vi "Test Copy Array To Image Pixel.vi"(8 "error in (no error)":errorcluster, 11 "Test Case In":refnum<class "Image.lvclass">) -> (0 "error out":errorcluster, 3 "Test Case Out":refnum<class "Image.lvclass">)   [LabVIEW 2020, in "g_ar_toolkit.test.lvlib" / "Image.lvclass"]
uses:
  Image.lvclass
  C:/Program Files (x86)/National Instruments/LabVIEW 2020/vi.lib/Astemes/LUnit/Test Case.lvclass
  g_ar_toolkit.common/Image Size (Integer).ctl
  <vilib>/Astemes/LUnit/Test Case.lvclass/Test Case.ctl
  g_ar_toolkit.image/New Image (ARGB).vi
  4993e8ee-a06a-463a-9684-69129f64d5ce.vi
  b5d9ff70-754c-4220-963e-cc8b9679940b.vi
  g_ar_toolkit.image/Copy Array to Image.vi
  g_ar_toolkit.image/Copy Array to Image (ARGB).vi
  g_ar_toolkit.image/New Image (ARGB).vi/3321fa97-f432-4e1e-8db9-a0df79aed21b.vi
  g_ar_toolkit.image/ARGB Colour to U32 Pixel Value.vi
  <vilib>/Astemes/LUnit/Append Pass Result.vi
  <vilib>/Astemes/LUnit/Append Fail Result.vi
  <vilib>/Astemes/LUnit/Describe Comparison.vi
  4993e8ee-a06a-463a-9684-69129f64d5ce.vi/9c5d11cd-9439-4240-a1ee-d9baace9c924.vi
  b5d9ff70-754c-4220-963e-cc8b9679940b.vi/9c5d11cd-9439-4240-a1ee-d9baace9c924.vi
  <vilib>/Astemes/LUnit/Run In UI.vi
  <vilib>/Utility/error.llb/Clear Errors.vi
  g_ar_toolkit.common/Module Path.vi
  <vilib>/Utility/error.llb/Error Cluster From Error Code.vi
  <vilib>/picture/pixmap.llb/Flatten Pixmap.vi
  <vilib>/Astemes/LUnit/Describe Variant.vi
  Image.lvclass/Image.ctl
  g_ar_toolkit.image/g_ar_toolkit.image.lvlib
  g_ar_toolkit.common/g_ar_toolkit.common.lvlib
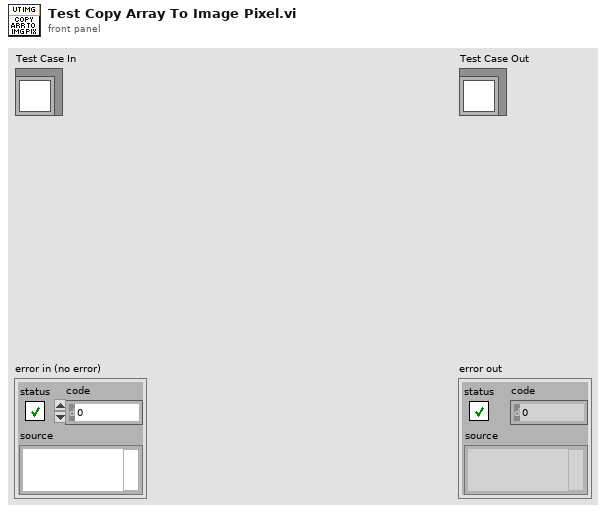
[diagram p1: front panel]
types:
  T1 = typedef "g_ar_toolkit.common.lvlib/Image Size (Integer).ctl" = cluster{"Width":u16, "Height":u16}
  T2 = typedef "g_ar_toolkit.image.lvlib/ARGB Image.ctl" = refnum<data-value>
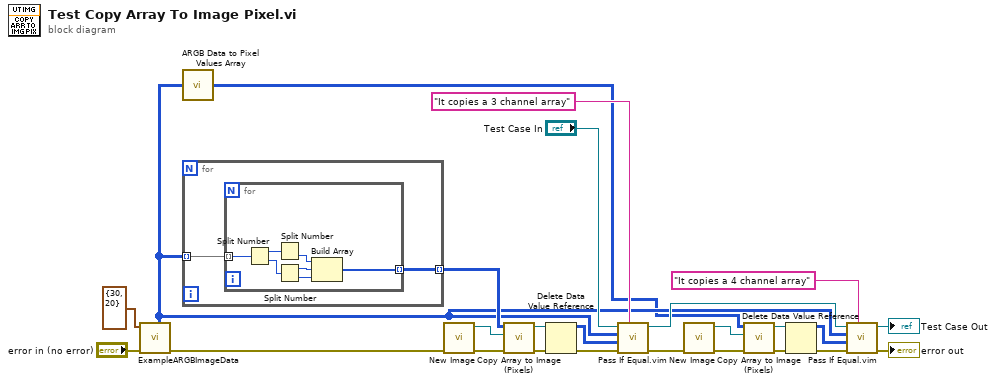
[diagram p0: block diagram]
diagram:
  n1 = call "ExampleARGBImageData.vi"("error in (no error)"="error in (no error)", "Image Size"=T1 {"Width"=30, "Height"=20}) -> ("error out"=w19:errorcluster, "ARGB Array Data"=w10:u32[][])  [unwired: 6 in, 2 out]
  n2 = call "ARGB Data to Pixel Values Array.vi"("ARGB Data"=w10) -> ("Pixel Values"=w3:u8[][][])
  n3 = for {
    tunnel: w10 -> [w27] mode=indexing
    tunnel: [w26] -> w16 mode=indexing
    n4 = for {
      tunnel: w27 -> [w34] mode=indexing
      tunnel: [w28] -> w26 mode=indexing
      n5 = Split Number(x=w34) -> (hi(x)=w32:u16, lo(x)=w33:u16)
      n6 = Split Number(x=w32) -> (lo(x)=w31:u8)  [unwired: 1 out]
      n7 = Split Number(x=w33) -> (hi(x)=w30:u8, lo(x)=w29:u8)
      n8 = Build Array(w31, w30, w29) -> (w28:u8[])
    }
  }
  n9 = call-poly "New Image.vi"("error in (no error)"=w19) -> ("error out"=w22:errorcluster, "New ARGB Image"=w21:T2)  [unwired: 9 in]
  n10 = call "Copy Array to Image (Pixels).vi"("error in (no error)"=w22, "ARGB Image Destination"=w21, "(A)RGB Pixels Data"=w16) -> ("error out"=w6:errorcluster, "ARGB Image Destination (Duplicate)"=w17:T2)  [unwired: 7 in]
  n11 = Delete Data Value Reference(data value reference=w17, error in=w6) -> (data value=w24:u32[][], error out=w23:errorcluster)
  n12 = call "Pass If Equal.vim"("Description"="It copies a 3 channel array", "error in (no error)"=w23, "Actual"=w24, "Expected"=w10, "LUnit Test Case In"="Test Case In") -> ("error out"=w12:errorcluster, "LUnit Test Case Out"=w11:refnum<class "Image.lvclass">)  [unwired: 5 in]
  n13 = call-poly "New Image.vi"("error in (no error)"=w12) -> ("error out"=w14:errorcluster, "New ARGB Image"=w13:T2)  [unwired: 9 in]
  n14 = call "Copy Array to Image (Pixels).vi"("error in (no error)"=w14, "ARGB Image Destination"=w13, "(A)RGB Pixels Data"=w3) -> ("error out"=w5:errorcluster, "ARGB Image Destination (Duplicate)"=w4:T2)  [unwired: 7 in]
  n15 = Delete Data Value Reference(data value reference=w4, error in=w5) -> (data value=w9:u32[][], error out=w8:errorcluster)
  n16 = call "Pass If Equal.vim"("Description"="It copies a 4 channel array", "error in (no error)"=w8, "Actual"=w9, "Expected"=w10, "LUnit Test Case In"=w11) -> ("error out"=→"error out":errorcluster, "LUnit Test Case Out"=→"Test Case Out":refnum<class "Image.lvclass">)  [unwired: 5 in]
